vi "Agilent VNA Read Start and Stop Frequencies.vi"(6 "Channel":i8=1 min=1 max=99 step=1, 7 "Agilent VNA":T1, 8 "error in (no error)":errorcluster, 11 "VISA Resource Name":refnum<visa-resource-name>) -> (0 "error out":errorcluster, 2 "Start/Stop Freqs, MHz":cluster{"Fstart":dbl, "Fstop":dbl}, 3 "dup VISA Resource Name":refnum<visa-resource-name>)   [LabVIEW 2011]
doc: "This VI for the HP8753B Network Analyzers reads the stimulus values. Except when performing log sweeps and freq list sweeps, this VI uses the start and stop values and the number of points to calcuate the stimulus values."
uses:
  TypeDefs/Agilent VNA Instrument Info.ctl
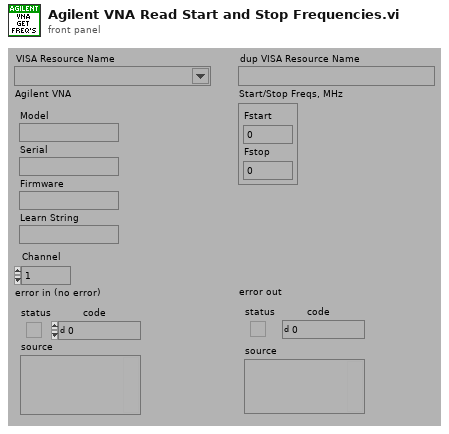
[diagram p1: front panel]
types:
  T1 = typedef "Agilent VNA Instrument Info.ctl" = cluster{"Model":string, "Serial":string, "Firmware":string, "Learn String":string}
  T2 = typedef "Agilent VNA Sweep Type.ctl" = enum32{"Linear Sweep", "Logarithmic Sweep", "Frequency List", "CW Time Sweep", "Power Sweep"}
  T3 = typedef "Agilent VNA Model.ctl" = enum16{"Not Supported", "8510X", "8719X", "8720X", "8722X", "8753X", "ENA", "PNA", "Field Fox"}
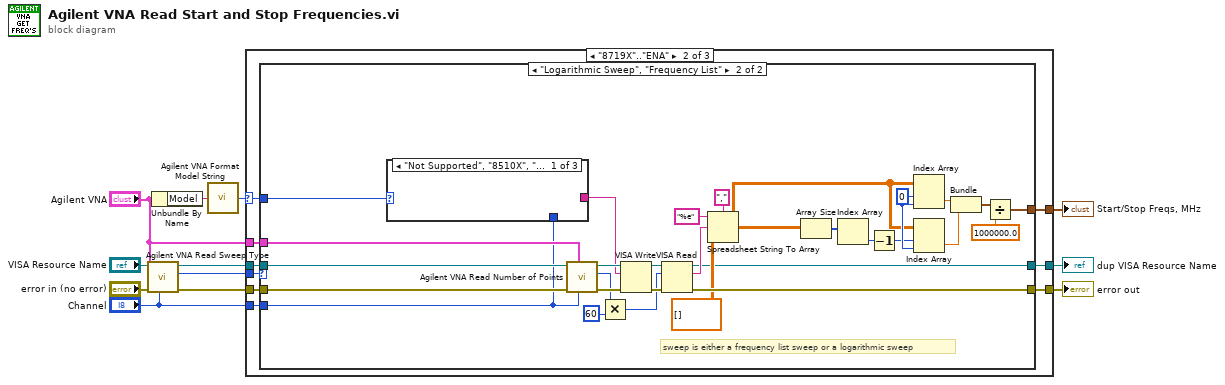
[diagram p0: block diagram]
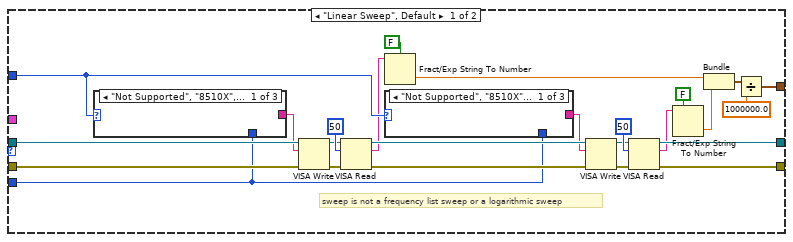
[diagram p3: hidden frame]
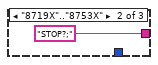
[diagram p4: hidden frame]
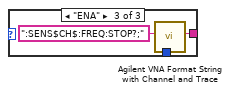
[diagram p5: hidden frame]
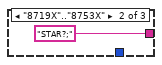
[diagram p6: hidden frame]
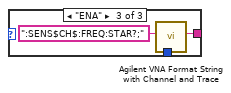
[diagram p7: hidden frame]
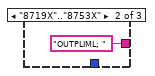
[diagram p8: hidden frame]
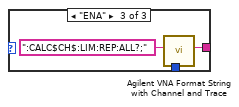
[diagram p9: hidden frame]
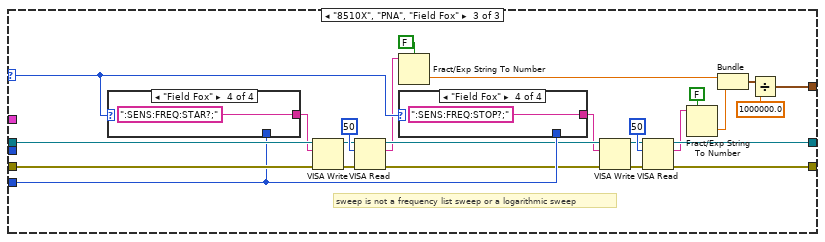
[diagram p10: hidden frame]
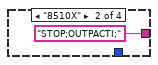
[diagram p12: hidden frame]
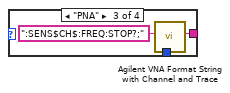
[diagram p13: hidden frame]
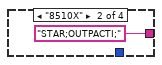
[diagram p15: hidden frame]
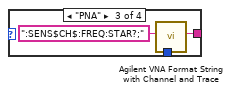
[diagram p16: hidden frame]
diagram:
  n1 = call "Agilent VNA Read Sweep Type.vi"("Channel"="Channel", "Agilent VNA"="Agilent VNA", "error in (no error)"="error in (no error)", "VISA Resource Name"="VISA Resource Name") -> ("error out"=w7:errorcluster, "Sweep Type"=w10:T2, "dup VISA Resource Name"=w8:refnum<visa-resource-name>)  [unwired: 5 out]
  n2 = Unbundle By Name("Agilent VNA") -> ("Model"=w3:string)
  n3 = call "Agilent VNA Format Model String.vi"("Model"=w3) -> ("Model"=w1:T3)
  n4 = case shown="\"8719X\"..\"ENA\"" w1 {
    selector: w1 -> [_ w15 w108]
    tunnel: [w13 w23 w114] -> w12
    tunnel: w10 -> [_ w22 _]
    tunnel: w8 -> [w14 w21 w113]
    tunnel: w7 -> [w13 w20 w112]
    tunnel: [_ w19 w111] -> w6
    tunnel: [w14 w18 w110] -> w5
    tunnel: "Channel" -> [_ w17 w109]
    tunnel: "Agilent VNA" -> [_ w16 _]
    frame "Not Supported" {
    }
    frame "8719X".."ENA" {
      n5 = case shown="\"Logarithmic Sweep\", \"Frequency List\"" w22 {
        tunnel: w21 -> [w47 w80]
        tunnel: w20 -> [w46 w78]
        tunnel: [w48 w83] -> w23
        tunnel: [w24 w57] -> w19
        tunnel: [w45 w63] -> w18
        tunnel: w15 -> [w44 w60]
        tunnel: w16 -> [_ w61]
        tunnel: w17 -> [w25 w58]
        frame "Linear Sweep", Default {
          # "sweep is not a frequency list sweep or a logarithmic sweep"
          n6 = case shown="\"Not Supported\", \"8510X\", \"PNA\", \"Field Fox\"" w44 {
            tunnel: [_ "STAR?;" w55] -> w27
            tunnel: w25 -> [_ _ w54]
            frame "Not Supported", "8510X", "PNA", "Field Fox" {
            }
            frame "8719X".."8753X" {
            }
            frame "ENA" {
              n7 = call "Agilent VNA Format String with Channel and Trace.vi"("Channel"=w54, "String"=":SENS$CH$:FREQ:STAR?;") -> ("String Out"=w55:string)  [unwired: 1 in, 6 out]
            }
          }
          n8 = VISA Write(VISA resource name=w47, write buffer=w27, error in (no error)=w46) -> (VISA resource name out=w34:refnum<visa-resource-name>, error out=w43:errorcluster)  [unwired: 1 out]
          n9 = VISA Read(VISA resource name=w34, byte count=u32 50, error in (no error)=w43) -> (VISA resource name out=w41:refnum<visa-resource-name>, read buffer=w39:string, error out=w40:errorcluster)  [unwired: 1 out]
          n10 = Fract/Exp String To Number(use system decimal point (T)=FALSE, string=w39) -> (number=w30:dbl)  [unwired: 3 out]
          n11 = case shown="\"Not Supported\", \"8510X\", \"PNA\", \"Field Fox\"" w44 {
            tunnel: [_ "STOP?;" w51] -> w26
            tunnel: w25 -> [_ _ w50]
            frame "Not Supported", "8510X", "PNA", "Field Fox" {
            }
            frame "8719X".."8753X" {
            }
            frame "ENA" {
              n12 = call "Agilent VNA Format String with Channel and Trace.vi"("Channel"=w50, "String"=":SENS$CH$:FREQ:STOP?;") -> ("String Out"=w51:string)  [unwired: 1 in, 6 out]
            }
          }
          n13 = VISA Write(VISA resource name=w41, write buffer=w26, error in (no error)=w40) -> (VISA resource name out=w35:refnum<visa-resource-name>, error out=w42:errorcluster)  [unwired: 1 out]
          n14 = VISA Read(VISA resource name=w35, byte count=u32 50, error in (no error)=w42) -> (VISA resource name out=w45:refnum<visa-resource-name>, read buffer=w38:string, error out=w48:errorcluster)  [unwired: 1 out]
          n15 = Fract/Exp String To Number(use system decimal point (T)=FALSE, string=w38) -> (number=w29:dbl)  [unwired: 3 out]
          n16 = Bundle(w30, w29) -> (w28:cluster{dbl, dbl})  [unwired: 1 out]
          n17 = Divide(x=w28, y=1000000.0) -> (x/y=w24:cluster{dbl, dbl})
        }
        frame "Logarithmic Sweep", "Frequency List" {
          w71 = 0 ("disabled index (col)")
          # "sweep is either a frequency list sweep or a logarithmic sweep"
          n18 = case shown="\"Not Supported\", \"8510X\", \"PNA\", \"Field Fox\"" w60 {
            tunnel: [_ "OUTPLIML; " w88] -> w59
            tunnel: w58 -> [_ _ w87]
            frame "Not Supported", "8510X", "PNA", "Field Fox" {
            }
            frame "8719X".."8753X" {
            }
            frame "ENA" {
              n19 = call "Agilent VNA Format String with Channel and Trace.vi"("Channel"=w87, "String"=":CALC$CH$:LIM:REP:ALL?;") -> ("String Out"=w88:string)  [unwired: 1 in, 6 out]
            }
          }
          n20 = call "Agilent VNA Read Number of Points.vi"("Channel"=w58, "Agilent VNA"=w61, "error in (no error)"=w78, "VISA Resource Name"=w80) -> ("error out"=w77:errorcluster, "Number Points"=w76:i32, "dup VISA Resource Name"=w79:refnum<visa-resource-name>)  [unwired: 5 out]
          n21 = Multiply(x=w76, y=60) -> (x*y=w81:i32)
          n22 = VISA Write(VISA resource name=w79, write buffer=w59, error in (no error)=w77) -> (VISA resource name out=w82:refnum<visa-resource-name>, error out=w85:errorcluster)  [unwired: 1 out]
          n23 = VISA Read(VISA resource name=w82, byte count=w81, error in (no error)=w85) -> (VISA resource name out=w63:refnum<visa-resource-name>, read buffer=w75:string, error out=w83:errorcluster)  [unwired: 1 out]
          n24 = Spreadsheet String To Array(delimiter (Tab)=",", format string="%e", spreadsheet string=w75, array type (2D Dbl)=dbl[][] []) -> (array=w62:dbl[][])
          n25 = Array Size(array=w62) -> (size(s)=w69:i32[])
          n26 = Index Array(array=w69) -> (element=w68:i32)  [unwired: 1 in]
          n27 = Decrement(x=w68) -> (x-1=w67:i32)
          n28 = Index Array(array=w62, index (row)=w71, index (col)=w71) -> (element=w70:dbl)
          n29 = Index Array(array=w62, index (row)=w67, index (col)=w71) -> (element=w66:dbl)
          n30 = Bundle(w70, w66) -> (w65:cluster{dbl, dbl})  [unwired: 1 out]
          n31 = Divide(x=w65, y=1000000.0) -> (x/y=w57:cluster{dbl, dbl})
        }
      }
    }
    frame "8510X", "PNA", "Field Fox" {
      # "sweep is not a frequency list sweep or a logarithmic sweep"
      n32 = case shown="\"Field Fox\"" w108 {
        tunnel: [_ "STAR;OUTPACTI;" w122 ":SENS:FREQ:STAR?;"] -> w91
        tunnel: w109 -> [_ _ w121 _]
        frame "Not Supported", "8719X".."ENA" {
        }
        frame "8510X" {
        }
        frame "PNA" {
          n33 = call "Agilent VNA Format String with Channel and Trace.vi"("Channel"=w121, "String"=":SENS$CH$:FREQ:STAR?;") -> ("String Out"=w122:string)  [unwired: 1 in, 6 out]
        }
        frame "Field Fox" {
        }
      }
      n34 = VISA Write(VISA resource name=w113, write buffer=w91, error in (no error)=w112) -> (VISA resource name out=w98:refnum<visa-resource-name>, error out=w107:errorcluster)  [unwired: 1 out]
      n35 = VISA Read(VISA resource name=w98, byte count=u32 50, error in (no error)=w107) -> (VISA resource name out=w105:refnum<visa-resource-name>, read buffer=w103:string, error out=w104:errorcluster)  [unwired: 1 out]
      n36 = Fract/Exp String To Number(use system decimal point (T)=FALSE, string=w103) -> (number=w94:dbl)  [unwired: 3 out]
      n37 = case shown="\"Field Fox\"" w108 {
        tunnel: [_ "STOP;OUTPACTI;" w117 ":SENS:FREQ:STOP?;"] -> w90
        tunnel: w109 -> [_ _ w116 _]
        frame "Not Supported", "8719X".."ENA" {
        }
        frame "8510X" {
        }
        frame "PNA" {
          n38 = call "Agilent VNA Format String with Channel and Trace.vi"("Channel"=w116, "String"=":SENS$CH$:FREQ:STOP?;") -> ("String Out"=w117:string)  [unwired: 1 in, 6 out]
        }
        frame "Field Fox" {
        }
      }
      n39 = VISA Write(VISA resource name=w105, write buffer=w90, error in (no error)=w104) -> (VISA resource name out=w99:refnum<visa-resource-name>, error out=w106:errorcluster)  [unwired: 1 out]
      n40 = VISA Read(VISA resource name=w99, byte count=u32 50, error in (no error)=w106) -> (VISA resource name out=w110:refnum<visa-resource-name>, read buffer=w102:string, error out=w114:errorcluster)  [unwired: 1 out]
      n41 = Fract/Exp String To Number(use system decimal point (T)=FALSE, string=w102) -> (number=w93:dbl)  [unwired: 3 out]
      n42 = Bundle(w94, w93) -> (w92:cluster{dbl, dbl})  [unwired: 1 out]
      n43 = Divide(x=w92, y=1000000.0) -> (x/y=w111:cluster{dbl, dbl})
    }
  }
  "dup VISA Resource Name" <- w5
  "error out" <- w12
  "Start/Stop Freqs, MHz" <- w6
